vi "Write outside terminal.vi"(5 "outside terminal":refnum<class "Terminal.lvclass">, 9 "FlatSequenceInnerTunnel in":refnum<class "FlatSequenceOuterTunnel.lvclass">) -> (3 "FlatSequenceInnerTunnel out":refnum<class "FlatSequenceOuterTunnel.lvclass">)   [LabVIEW 2014, in "Raspberry Pi Compatible Compiler for LabVIEW.lvlib" / "FlatSequenceOuterTunnel.lvclass"]
uses:
  FlatSequenceOuterTunnel.lvclass
  Terminal/Terminal.lvclass
  FlatSequenceOuterTunnel.lvclass/FlatSequenceOuterTunnel.ctl
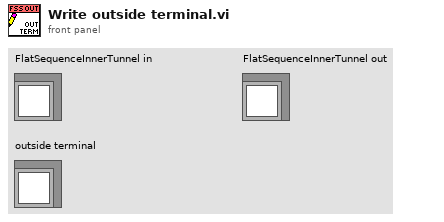
[diagram p1: front panel]
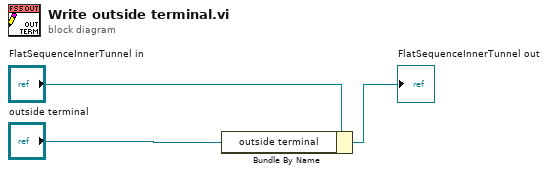
[diagram p0: block diagram]
diagram:
  n1 = Bundle By Name(cluster="FlatSequenceInnerTunnel in", "outside terminal"="outside terminal") -> (→"FlatSequenceInnerTunnel out":refnum<class "FlatSequenceOuterTunnel.lvclass">)
